vi "limit_cursors.vi"(8 "error in (no error)":errorcluster, 11 "ColorOverlay in":refnum<class "ColorOverlay.lvclass">) -> (0 "error out":errorcluster, 3 "ColorOverlay out":refnum<class "ColorOverlay.lvclass">)   [LabVIEW 2010, in "ColorOverlay.lvclass"]
uses:
  ColorOverlay.lvclass
  ColorOverlay.lvclass/ColorOverlay.ctl
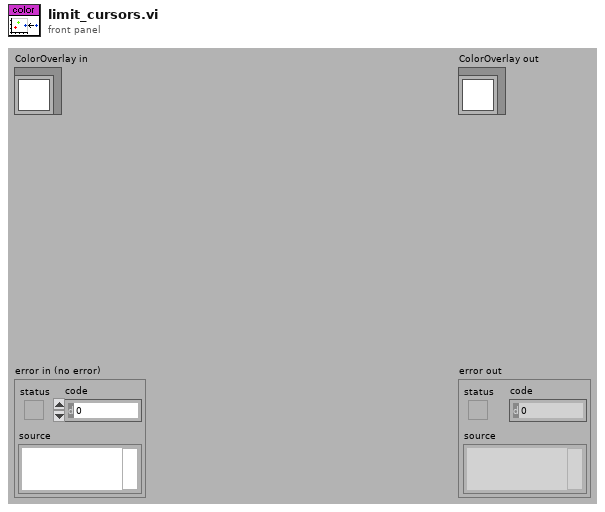
[diagram p1: front panel]
types:
  T1 = typedef "ColorOverlay.lvclass/cursor_cluster.ctl" = cluster{"cursor position":dbl[]}
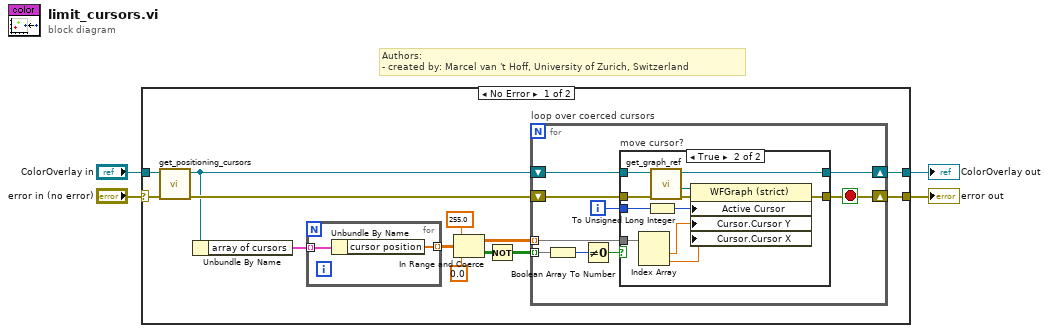
[diagram p0: block diagram]
diagram:
  # "Authors: \n- created by: Marcel van 't Hoff, University of Zurich, Switzerland"
  n1 = case shown="No Error" "error in (no error)" {
    selector: "error in (no error)" -> [w17 w43]
    tunnel: [w11 w43] -> w3
    tunnel: [w10 w42] -> w1
    tunnel: "ColorOverlay in" -> [w16 w42]
    frame No Error {
      n2 = call-dynamic "get_positioning_cursors.vi"("error in (no error)"=w17, "ColorOverlay in"=w16) -> ("error out"=w12:errorcluster, "ColorOverlay out"=w7:refnum<class "ColorOverlay.lvclass">)  [unwired: 8 in]
      n3 = Unbundle By Name(w7) -> ("array of cursors"=w6:T1[])
      n4 = for {
        tunnel: w6 -> [w19] mode=indexing
        tunnel: [w18] -> w5 mode=indexing
        n5 = Unbundle By Name(w19) -> ("cursor position"=w18:dbl[])
      }
      n6 = In Range and Coerce(upper limit=255.0, x=w5, lower limit=0.0) -> (coerced(x)=w9:dbl[][], In Range?=w13:bool[][])
      n7 = Not(x=w13) -> (.not. x?=w8:bool[][])
      n8 = for "loop over coerced cursors" {
        tunnel: w9 -> [w23] mode=indexing
        tunnel: w8 -> [w28] mode=indexing
        shift-right: [w20] -> w11
        shift-left: w12 -> [w24]
        shift-right: [w22] -> w10
        shift-left: w7 -> [w25]
        i -> [w21]
        stop <- w20 stop-if-true
        n9 = Boolean Array To Number(Boolean array=w28) -> (number=w27:u32)
        n10 = Not Equal To 0?(x=w27) -> (x != 0?=w26:bool)
        n11 = case "move cursor?" shown="True" w26 {
          tunnel: w25 -> [w29 w41]
          tunnel: w24 -> [w30 w40]
          tunnel: w23 -> [_ w37]
          tunnel: [w30 w36] -> w20
          tunnel: [w29 w35] -> w22
          tunnel: w21 -> [_ w31]
          frame False {
          }
          frame True {
            n12 = Index Array(array=w37) -> (element #1=w33:dbl, element #2=w32:dbl)  [unwired: 2 in]
            n13 = To Unsigned Long Integer(number=w31) -> (unsigned 32bit integer=w34:u32)
            n14 = call-dynamic "get_graph_ref.vi"("error in (no error)"=w40, "ColorOverlay in"=w41) -> ("error out"=w38:errorcluster, "graph ref"=w39:refnum<vi>, "ColorOverlay out"=w35:refnum<class "ColorOverlay.lvclass">)  [unwired: 7 in]
            n15 = property class="WFGraph (strict)"(reference=w39, error in=w38, "Active Cursor"=w34, "Cursor.Cursor Y"=w33, "Cursor.Cursor X"=w32) -> (error out=w36:errorcluster)  [unwired: 1 out]
          }
        }
      }
    }
    frame Error {
    }
  }
  "error out" <- w3
  "ColorOverlay out" <- w1
